vi "Feed Ball to Shooter.vi"(1 "Execute":bool=TRUE) -> (4 "Done Executing":bool)   [LabVIEW 2012]
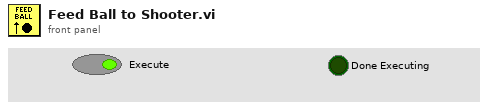
[diagram p1: front panel]
types:
  T1 = typedef "WPI_MotorControlDeviceRef.ctl" = cluster{"DeviceStatus":errorcluster, "Type":enum16{"PWM", "CAN"}, "PWM":cluster{"Digital Module":T2, "PWM Channel":T3, "DeadBand":T4}, "CAN":cluster{"Device Number":u8, "Control Mode":T5, "Semaphore":T6, "Max Vout":dbl}, "Invert":bool, "TransformRef":T7, "InvTransformRef":T7}
  T2 = typedef "FPGA_TypedefDigitalModule.ctl" = enum16{"Digital Module 1", "Digital Module 2"}
  T3 = typedef "FPGA_DIOPWMChannel.ctl" = enum8{"PWM 1", "PWM 2", "PWM 3", "PWM 4", "PWM 5", "PWM 6", "PWM 7", "PWM 8", "PWM 9", "PWM 10", "Invalid"}
  T4 = typedef "WPI_PWMDeadband.ctl" = cluster{"Name":string, "maxPositivePwm":i32, "minPositivePwm":i32, "centerPwm":i32, "maxNegativePwm":i32, "minNegativePwm":i32, "angularRange":u16}
  T5 = typedef "WPI_CANJaguar_ControlMode.ctl" = enum8{"Percent VBus", "Current", "Speed", "Position", "Voltage"}
  T6 = typedef "Semaphore RefNum" = refnum<k1>
  T7 = typedef "WPI_PWMTransform_ConPane.ctl" = refnum<vi>
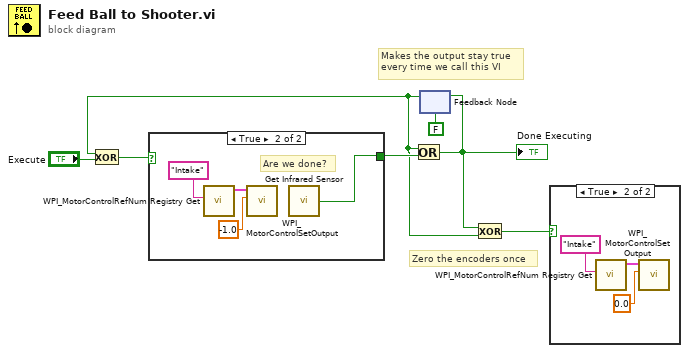
[diagram p0: block diagram]
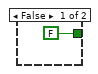
[diagram p3: hidden frame]
diagram:
  # "Zero the encoders once"
  # "Makes the output stay true\nevery time we call this VI"
  n1 = feedback #1(FALSE) -> (w2:bool)
  n2 = Exclusive Or(1:"Execute", 2:w2) -> (0:w7:bool)
  n3 = case shown="True" w7 {
    tunnel: [FALSE w12] -> w5
    frame False {
    }
    frame True {
      # "Are we done?"
      n4 = call <vilib>:"WPI_MotorControlRefNum Registry Get.vi"("refnum name"="Intake") -> ("MotorControlDevRef"=w10:T1)  [unwired: 9 in, 1 out]
      n5 = call <vilib>:"WPI_MotorControlSetOutput.vi"("Output"=-1.0, "MotorControlDevRef"=w10) -> ()  [unwired: 7 in, 3 out]
      n6 = call "Get Infrared Sensor.vi"() -> ("Laser Broken?"=w12:bool)
    }
  }
  n7 = Or(x=w2, y=w5) -> (x .or. y?=w1:bool)
  "Done Executing" <- w1
  n8 = feedback-in #1(w1) -> ()
  n9 = Exclusive Or(1:w2, 2:w1) -> (0:w3:bool)
  n10 = case shown="True" w3 {
    frame False {
    }
    frame True {
      n11 = call <vilib>:"WPI_MotorControlRefNum Registry Get.vi"("refnum name"="Intake") -> ("MotorControlDevRef"=w14:T1)  [unwired: 9 in, 1 out]
      n12 = call <vilib>:"WPI_MotorControlSetOutput.vi"("Output"=0.0, "MotorControlDevRef"=w14) -> ()  [unwired: 7 in, 3 out]
    }
  }
